vi "2021T01096(LABVIEW FILE).vi"() -> ()   [LabVIEW 2024]
uses:
  Program Files (x86)/National Instruments/Control 1.ctl
  Program Files (x86)/National Instruments/Control 2.ctl
  <vilib>/Instr/_visa.llb/VISA Configure Serial Port (Instr).vi
panel:
  out "INDICATOR":bool
  out "INDICATOR":bool
  out "HUMIDITY WAVEFORM GRAPH":dbl(graph)
  out "TEMPERATURE WAVEFORM GRAPH":dbl(graph)
  out "DISTANCE WAVEFORM GRAPH":dbl(graph)
  out "GAS VALUE WAVEFORM GRAPH":dbl(graph)
  out "BUZZER INDICATOR":bool
  in  "BUZZER CONTROL":bool
  out "NORMAL":bool
  out "COLD":bool
  out "WARM":bool
  out "MEDIUM":bool
  out "LOW":bool
  out "HIGH":bool
  in  "STOP SESSION":bool
  out "SENSOR VALUES":string
  in  "BAUD RATE":u32=10000
  out "HUMIDITY":dbl(slide) scale=0.0..150.0
  out "DISTANCE":dbl(slide) scale=0.0..200.0
  out "TEMPARATURE VALUE":T1 scale=0.0..50.0
  out "GAS VALUE":T2 scale=0.0..600.0
  in  "VISA resource name":refnum<visa-resource-name>
  # "IA 3204 – Data Acquisition Systems Project"
  # "CONTROL PANEL"
  # "DATA INTERFACE"
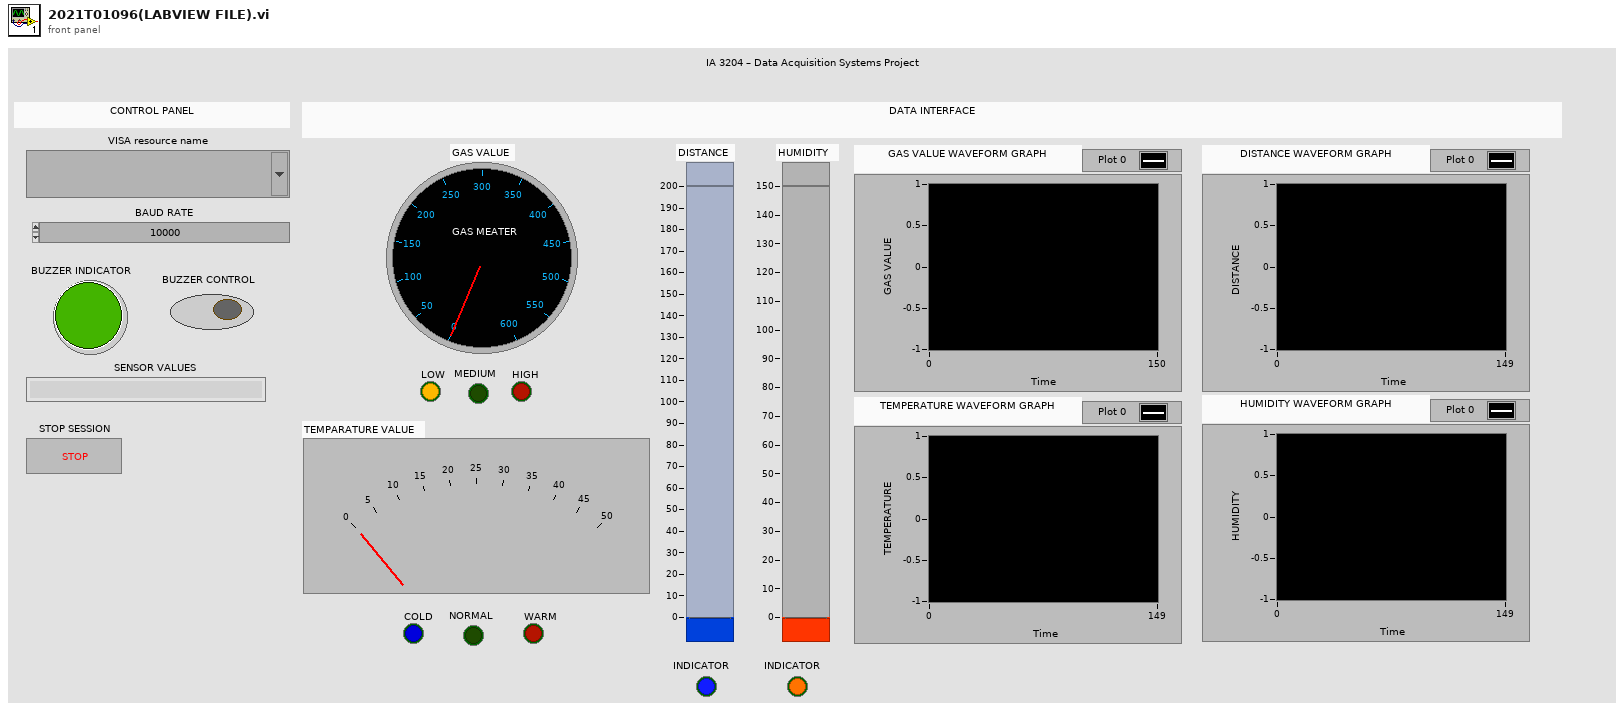
[diagram p1: front panel]
types:
  T1 = typedef "Control 2.ctl" = dbl
  T2 = typedef "Control 1.ctl" = dbl
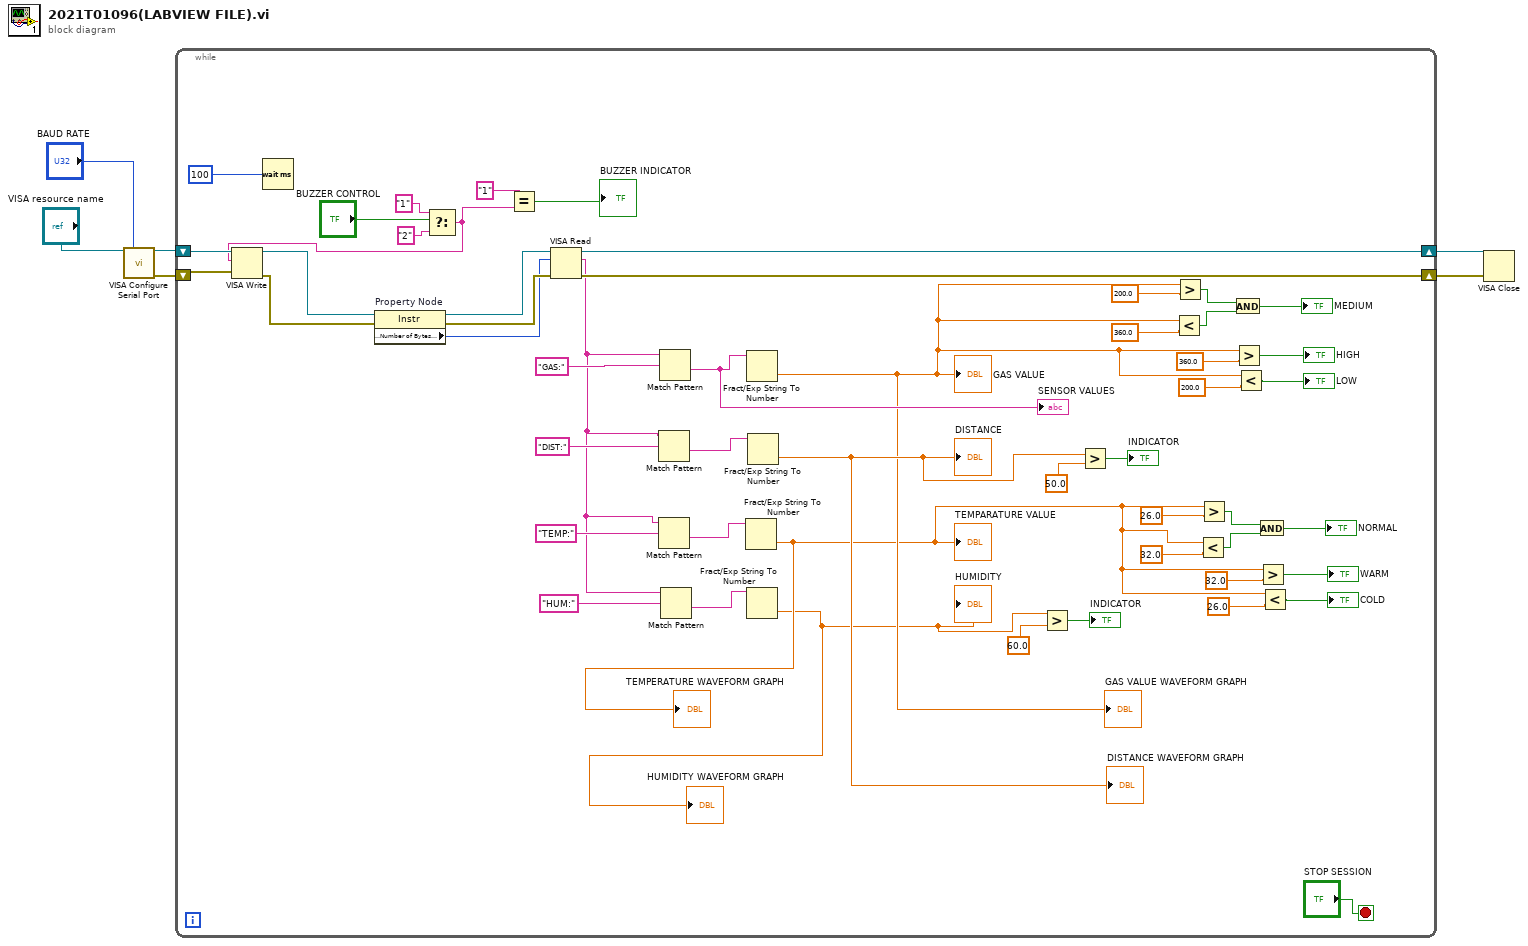
[diagram p0: block diagram]
diagram:
  n1 = call-poly "VISA Configure Serial Port"("VISA resource name"="VISA resource name", "timeout (10sec)"="BAUD RATE") -> ("VISA resource name out"=w5:refnum<visa-resource-name>, "error out"=w4:errorcluster)  [unwired: 12 in]
  n2 = while {
    shift-right: [w51] -> w3
    shift-left: w5 -> [w58]
    shift-right: [w50] -> w2
    shift-left: w4 -> [w57]
    stop <- "STOP SESSION" stop-if-true
    n3 = Wait (ms)(milliseconds to wait=u32 100) -> ()  [unwired: 1 out]
    n4 = Select(t="1", s="BUZZER CONTROL", f="2") -> (s? t:f=w17:string)
    n5 = VISA Write(VISA resource name=w58, write buffer=w17, error in (no error)=w57) -> (VISA resource name out=w56:refnum<visa-resource-name>, error out=w55:errorcluster)  [unwired: 1 out]
    n6 = property on="Property Node" class="Instr"(reference=w56, error in=w55) -> (reference out=w54:refnum<visa-resource-name>, error out=w53:errorcluster, "Serial Settings:Number of Bytes at Serial Port"=w52:u32)
    n7 = Equal?(x="1", y=w17) -> (x = y?=→"BUZZER INDICATOR":bool)
    n8 = VISA Read(VISA resource name=w54, byte count=w52, error in (no error)=w53) -> (VISA resource name out=w51:refnum<visa-resource-name>, read buffer=w40:string, error out=w50:errorcluster)  [unwired: 1 out]
    n9 = Match Pattern(string=w40, regular expression="DIST:") -> (after substring=w15:string)  [unwired: 1 in, 3 out]
    n10 = Match Pattern(string=w40, regular expression="TEMP:") -> (after substring=w43:string)  [unwired: 1 in, 3 out]
    n11 = Match Pattern(string=w40, regular expression="GAS:") -> (after substring=w44:string)  [unwired: 1 in, 3 out]
    "SENSOR VALUES" <- w44
    n12 = Match Pattern(string=w40, regular expression="HUM:") -> (after substring=w42:string)  [unwired: 1 in, 3 out]
    n13 = Fract/Exp String To Number(string=w43) -> (number=w8:dbl)  [unwired: 3 in, 1 out]
    "TEMPARATURE VALUE" <- w8
    "TEMPERATURE WAVEFORM GRAPH" <- w8
    n14 = Fract/Exp String To Number(string=w44) -> (number=w9:dbl)  [unwired: 3 in, 1 out]
    "GAS VALUE" <- w9
    "GAS VALUE WAVEFORM GRAPH" <- w9
    n15 = Fract/Exp String To Number(string=w42) -> (number=w7:dbl)  [unwired: 3 in, 1 out]
    "HUMIDITY" <- w7
    "HUMIDITY WAVEFORM GRAPH" <- w7
    n16 = Fract/Exp String To Number(string=w15) -> (number=w10:dbl)  [unwired: 3 in, 1 out]
    "DISTANCE" <- w10
    "DISTANCE WAVEFORM GRAPH" <- w10
    n17 = Greater?(x=w7, y=60.0) -> (0:→"INDICATOR":bool)
    n18 = Greater?(x=w10, y=50.0) -> (0:→"INDICATOR":bool)
    n19 = Less?(x=w9, y=360.0) -> (x < y?=w33:bool)
    n20 = Greater?(x=w9, y=200.0) -> (0:w34:bool)
    n21 = Less?(x=w8, y=32.0) -> (x < y?=w24:bool)
    n22 = Greater?(x=w8, y=26.0) -> (0:w25:bool)
    n23 = And(x=w34, y=w33) -> (x .and. y?=→"MEDIUM":bool)
    n24 = Greater?(x=w9, y=360.0) -> (0:→"HIGH":bool)
    n25 = Less?(x=w9, y=200.0) -> (x < y?=→"LOW":bool)
    n26 = And(x=w25, y=w24) -> (x .and. y?=→"NORMAL":bool)
    n27 = Greater?(x=w8, y=32.0) -> (0:→"WARM":bool)
    n28 = Less?(x=w8, y=26.0) -> (x < y?=→"COLD":bool)
  }
  n29 = VISA Close(VISA resource name=w3, error in (no error)=w2) -> ()  [unwired: 1 out]
